vi "3 Optical Motion (Eyes Looking For Geometry).vi"() -> ()   [LabVIEW 2012]
doc: "This example shows how to use the Lucas Kanade Pyramid motion estimation VI to track features in a sequence of images in NI Vision. The VI reads the frames from an AVI file and tracks user specified features in the image from frame to frame."
uses:
  Controls/EyeOptionsCluster.ctl
  <vilib>/userdefined/High Color/IMAQdx.ctl
  <vilib>/vision/Pattern Matching.llb/IMAQ Curve Parameters.ctl
  <vilib>/vision/driver/NI_Vision_Acquisition_Software.lvlib
  <vilib>/vision/NI_Vision_Development_Module.lvlib
panel:
  in  "Eye Options":T1={"Eye Size"=1.0, "Overlay Eyes?"=TRUE, "Eye Tracking?"=TRUE} {"Eye Size" items=["Small"=0.5, "Medium"=1, "Large"=2]}
  in  "Select Points":bool caption="Click on the image and select the points to track. Press the <Ctrl> key while selecting  multiple points. Press the  \"Select Points\" button after  all points have been selected."
  out "Image":T2(plugin-control)
  in  "Stop":bool
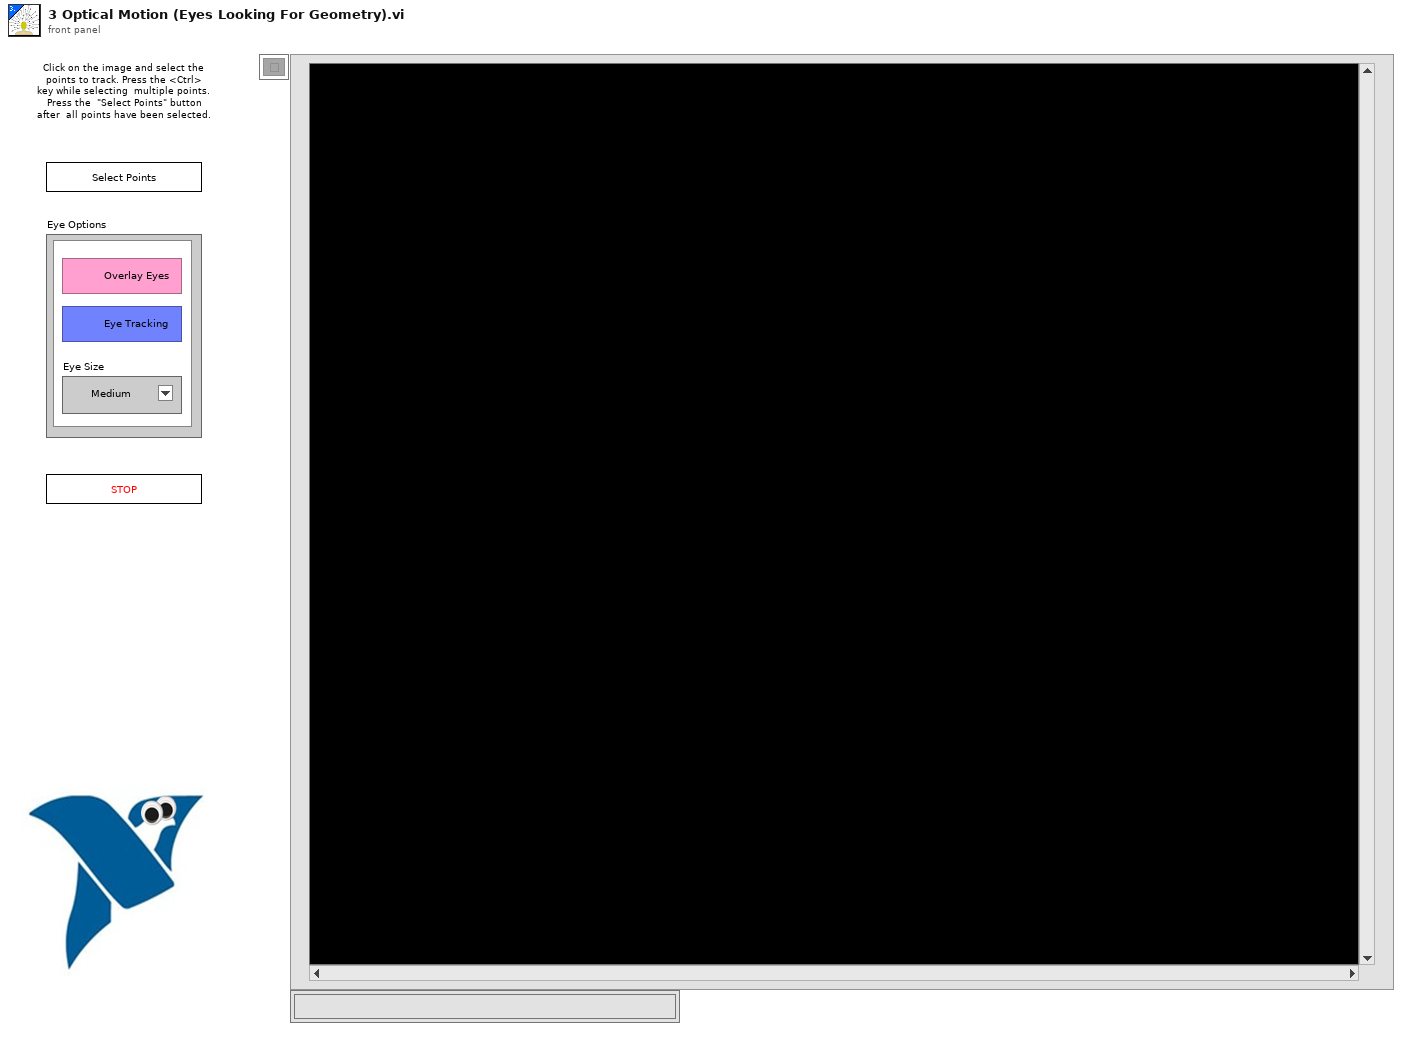
[diagram p1: front panel]
types:
  T1 = typedef "EyeOptionsCluster.ctl" = cluster{"Eye Size":sgl, "Overlay Eyes?":bool, "Eye Tracking?":bool}
  T2 = typedef "IMAQ Image.ctl" = refnum<image>
  T3 = typedef "IMAQ Point" = cluster{"X":sgl, "Y":sgl}
  T4 = typedef "IMAQ Curve Parameters.ctl" = cluster{"Extraction Mode":u32, "Edge Threshold":i32, "Edge Filter Size":u32, "Min Length":i32, "Row Search Step Size":i32, "Col Search Step Size":i32, "Max Endpoint Gap":i32, "Closed":bool, "Subpixel":bool}
  T5 = cluster{"Rotation":bool, "Scale":bool, "Occlusion":bool, "Reserved":bool, "Reserved":bool, "Reserved":bool}
  T6 = typedef "IMAQdx.ctl" = refnum<k21>
  T7 = cluster{"Level":i32, "maxiteration":i32, "windowsize":i32, "threshold":dbl}
  T8 = cluster{"Left":i32, "Top":i32, "Right":i32, "Bottom":i32}
  T9 = typedef "IMAQ GM Match Report.ctl" = cluster{"Position":cluster{"x":sgl, "y":sgl}, "Angle":sgl, "Scale":sgl, "Score":sgl, "Bounding Box":cluster{"x":sgl, "y":sgl}[], "Contrast Reversed":bool, "Occlusion %":sgl, "Template Target Curve Score":sgl, "Target Template Curve Score":sgl, "Correlation Score":sgl}
  T10 = cluster{"Global Rectangle":i32[], "Contours":cluster{"Contour Type":u32, "ROI Type":u32, "Points":i32[]}[]}
  T11 = typedef "ROI Descriptor" = cluster{"Global Rectangle":i32[], "Contours":cluster{"ID":enum32{"External", "Internal"}, "Type":u32, "Coordinates":i32[]}[]}
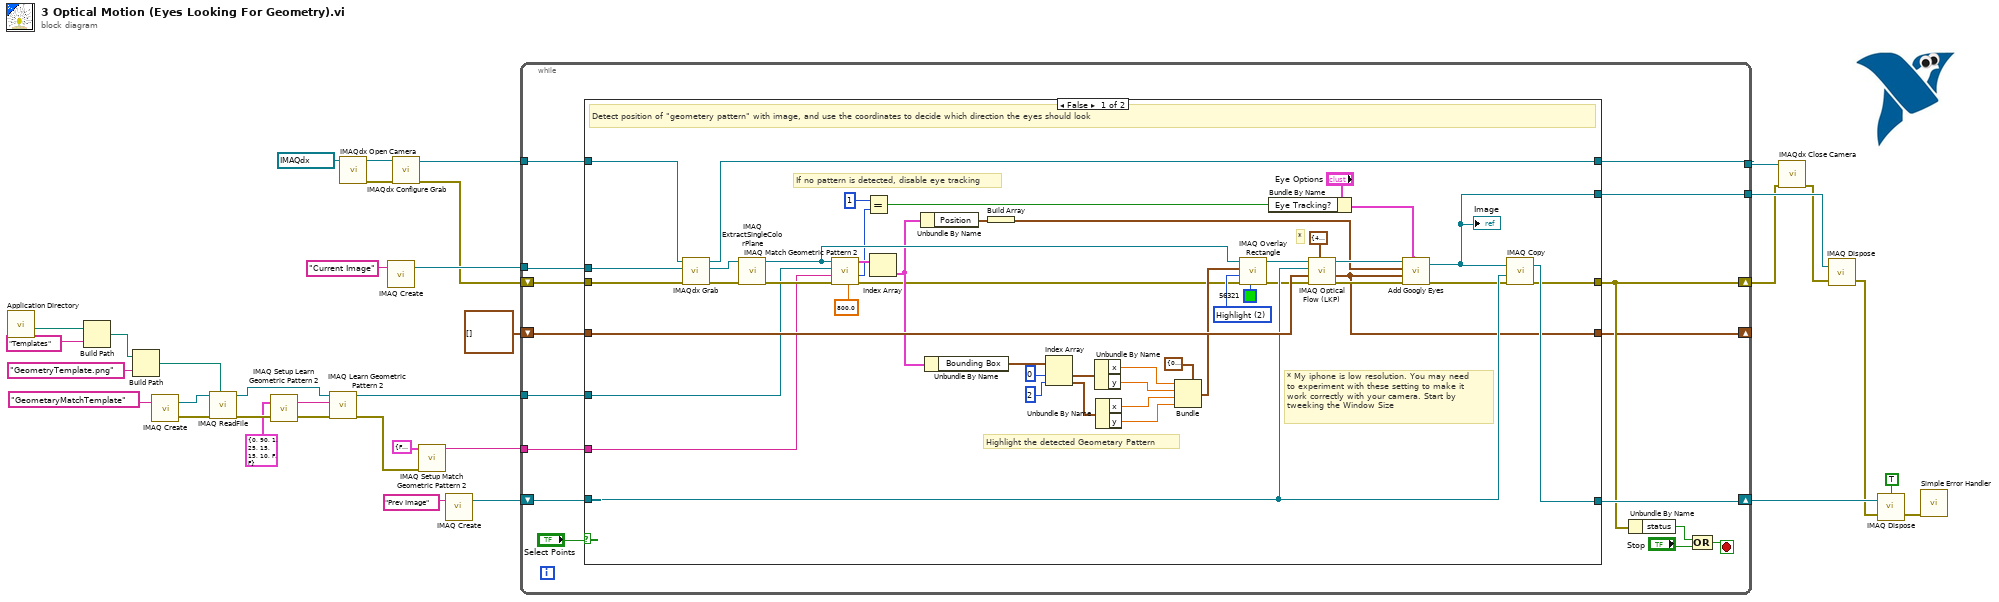
[diagram p0: block diagram]
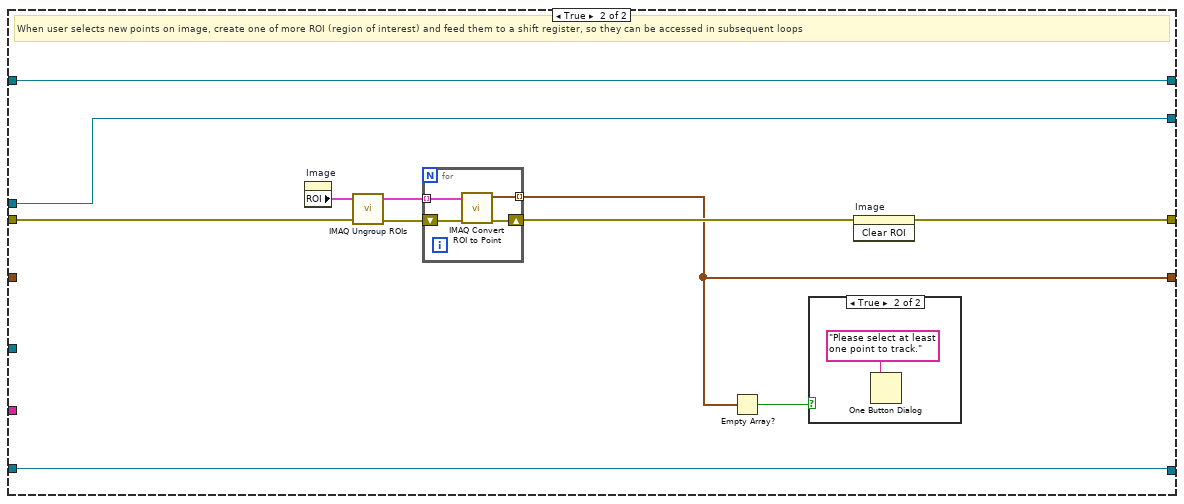
[diagram p2: hidden frame]
diagram:
  n1 = call <vilib>:"Application Directory.vi"() -> ("Application Directory"=w4:path)
  n2 = Build Path(base path=w4, name or relative path="Templates") -> (appended path=w3:path)
  n3 = Build Path(base path=w3, name or relative path="GeometryTemplate.png") -> (appended path=w19:path)
  n4 = call "IMAQ Create"("Image Name"="GeometaryMatchTemplate") -> ("New Image"=w15:T2, "error out"=w17:errorcluster)  [unwired: 4 in]
  n5 = call "IMAQ ReadFile"("File Path"=w19, "error in (no error)"=w17, "Image"=w15) -> ("error out"=w13:errorcluster, "Image Out"=w12:T2)  [unwired: 4 in, 3 out]
  n6 = call "IMAQ Setup Learn Geometric Pattern 2"("error in (no error)"=w13, "Curve Parameters"=T4 {"Extraction Mode"=0, "Edge Threshold"=90, "Edge Filter Size"=1, "Min Length"=25, "Row Search Step Size"=15, "Col Search Step Size"=15, "Max Endpoint Gap"=10, "Closed"=FALSE, "Subpixel"=FALSE}) -> ("error out"=w11:errorcluster, "Learn Geometric Pattern 2 Setup Data"=w9:string)
  n7 = call "IMAQ Learn Geometric Pattern 2"("error in (no error)"=w11, "Learn Geometric Pattern 2 Setup Data"=w9, "Template Image"=w12) -> ("error out"=w7:errorcluster, "Template Image Out"=w10:T2)  [unwired: 7 in]
  n8 = call <vilib>:"IMAQdx Open Camera.vi"("Session In"=T6 "iPhone") -> ("error out"=w27:errorcluster, "Session Out"=w28:T6)  [unwired: 9 in]
  n9 = call "IMAQ Create"("Image Name"="Current Image") -> ("New Image"=w34:T2)  [unwired: 3 in, 2 out]
  n10 = call <vilib>:"IMAQdx Configure Grab.vi"("error in"=w27, "Session In"=w28) -> ("error out"=w21:errorcluster, "Session Out"=w22:T6)  [unwired: 8 in]
  n11 = call "IMAQ Setup Match Geometric Pattern 2"("error in (no error)"=w7, "Match Mode"=T5 {"Rotation"=FALSE, "Scale"=TRUE, "Occlusion"=FALSE, "Reserved"=FALSE, "Reserved"=FALSE, "Reserved"=FALSE}) -> ("Match Geometric Pattern 2 Setup Data"=w8:string)  [unwired: 8 in, 1 out]
  n12 = call "IMAQ Create"("Image Name"="Prev Image") -> ("New Image"=w20:T2)  [unwired: 3 in, 2 out]
  n13 = while {
    tunnel: w34 -> [w41]
    shift-right: [w46] -> w31
    shift-left: w20 -> [w48]
    shift-right: [w43] -> _
    shift-left: T3[] [] ("Feature Points Out") -> [w44]
    shift-right: [w45] -> w26
    shift-left: w21 -> [w51]
    tunnel: [w40] -> w32
    tunnel: w22 -> [w39]
    tunnel: [w38] -> w30
    tunnel: w10 -> [w37]
    tunnel: w8 -> [w36]
    stop <- w49 stop-if-true
    n14 = case shown="False" "Select Points" {
      tunnel: w51 -> [w97 w103]
      tunnel: w41 -> [w96 w102]
      tunnel: w48 -> [w90 w108]
      tunnel: [w95 w108] -> w46
      tunnel: [w94 w99] -> w45
      tunnel: w44 -> [w93 _]
      tunnel: [w84 w101] -> w43
      tunnel: [w83 w102] -> w40
      tunnel: w39 -> [w92 w98]
      tunnel: [w91 w98] -> w38
      tunnel: w37 -> [w80 _]
      tunnel: w36 -> [w79 _]
      frame False {
        w74 = u32 2 items=["Frame", "Fill", "Highlight"] ("Drawing Mode (Frame)")
        # "*"
        # "* My iphone is low resolution. You may need\nto experiment with these setting to make it\nwork correctly with your camera. Start by \ntweeking the Window Size"
        # "Highlight the detected Geometary Pattern"
        # "If no pattern is detected, disable eye tracking"
        # "Detect position of \"geometery pattern\" with image, and use the coordinates to decide which direction the eyes should look"
        n15 = call <vilib>:"IMAQdx Grab.vi"("error in"=w97, "Image In"=w96, "Session In"=w92) -> ("error out"=w87:errorcluster, "Image Out"=w88:T2, "Session Out"=w91:T6)  [unwired: 5 in, 1 out]
        n16 = call "IMAQ ExtractSingleColorPlane"("error in (no error)"=w87, "Image Src"=w88) -> ("error out"=w81:errorcluster, "Image Dst Out"=w73:T2)  [unwired: 8 in]
        n17 = call "IMAQ Match Geometric Pattern 2"("Minimum Match Score"=sgl 800.0, "error in (no error)"=w81, "Match Geometric Pattern 2 Setup Data"=w79, "Template Image"=w80, "Image"=w73) -> ("error out"=w58:errorcluster, "Number of Matches"=w55:i32, "Matches (pixel)"=w77:T9[])  [unwired: 3 in, 1 out]
        n18 = Equal?(x=1, y=w55) -> (x = y?=w53:bool)
        n19 = Index Array(array=w77) -> (element=w64:T9)  [unwired: 1 in]
        n20 = Unbundle By Name(w64) -> ("Position"=w76:cluster{"x":sgl, "y":sgl})
        n21 = Unbundle By Name(w64) -> ("Bounding Box"=w69:cluster{"x":sgl, "y":sgl}[])
        n22 = Build Array(w76) -> (w75:cluster{"x":sgl, "y":sgl}[])
        n23 = Index Array(array=w69, index #1=0 ("index"), index #2=2 ("index")) -> (element #1=w66:cluster{"x":sgl, "y":sgl}, element #2=w65:cluster{"x":sgl, "y":sgl})
        n24 = Unbundle By Name(w66) -> ("x"=w63:sgl, "y"=w62:sgl)
        n25 = Unbundle By Name(w65) -> ("x"=w61:sgl, "y"=w60:sgl)
        n26 = Bundle(cluster=T8 {"Left"=0, "Top"=0, "Right"=0, "Bottom"=0} ("Rectangle"), "Left"=w63, "Top"=w62, "Right"=w61, "Bottom"=w60) -> (w70:T8)
        n27 = call "IMAQ Overlay Rectangle"("Color"=u32 56321, "error in (no error)"=w58, "Drawing Mode (Frame)"=w74, "Rectangle"=w70, "Image"=w73) -> ("error out"=w59:errorcluster, "Image Out"=w72:T2)  [unwired: 5 in]
        n28 = Bundle By Name(cluster="Eye Options", "Eye Tracking?"=w53) -> (w52:T1)
        n29 = call "IMAQ Optical Flow (LKP)"("Options"=T7 {"Level"=4, "maxiteration"=5, "windowsize"=15, "threshold"=0.01} ("Optical Flow Options"), "error in (no error)"=w59, "Feature Points In"=w93, "Previous Frame"=w90, "Current Frame"=w72) -> ("error out"=w86:errorcluster, "Feature Points Out"=w84:cluster{"X":sgl, "Y":sgl}[], "Current Frame Out (dup)"=w82:T2)  [unwired: 1 in, 3 out]
        n30 = call "Add Googly Eyes.vi"("Eye Options"=w52, "error in (no error)"=w86, "Eye Coordinates"=w84, "Feature Coordinates"=w75, "ImageRef In"=w82) -> ("error out"=w89:errorcluster, "ImageRef out"=w83:T2)  [unwired: 5 in]
        "Image" <- w83
        n31 = call "IMAQ Copy"("error in (no error)"=w89, "Image Dst"=w90, "Image Src"=w83) -> ("error out"=w94:errorcluster, "Image Dst Out"=w95:T2)  [unwired: 3 out]
      }
      frame True {
        # "When user selects new points on image, create one of more ROI (region of interest) and feed them to a shift register, so they can be accessed in subsequent loops"
        n32 = property on="Image" class="ImageControl"() -> ("ROI"=w107:T10)  [unwired: 2 in, 2 out]
        n33 = call "IMAQ Ungroup ROIs"("error in (no error)"=w103, "ROI Descriptor"=w107) -> ("error out"=w106:errorcluster, "ROI Descriptors out"=w105:T11[])  [unwired: 2 out]
        n34 = for {
          shift-right: [w110] -> w104
          shift-left: w106 -> [w113]
          tunnel: w105 -> [w112] mode=indexing
          tunnel: [w111] -> w101 mode=indexing
          n35 = call "IMAQ Convert ROI to Point"("error in (no error)"=w113, "ROI Descriptor"=w112) -> ("error out"=w110:errorcluster, "Point"=w111:T3)  [unwired: 7 out]
        }
        n36 = Empty Array?(array=w101) -> (empty?=w100:bool)
        n37 = case shown="True" w100 {
          frame False {
          }
          frame True {
            n38 = One Button Dialog(message="Please select at least one point to track.") -> ()  [unwired: 2 out]
          }
        }
        n39 = invoke on="Image" class="ImageControl" method="Clear ROI"(error in=w104) -> (error out=w99:errorcluster)  [unwired: 2 in, 2 out]
      }
    }
    n40 = Unbundle By Name(w45) -> ("status"=w47:bool)
    n41 = Compound Arithmetic op=OR(w47, "Stop") -> (w49:bool)
  }
  n42 = call <vilib>:"IMAQdx Close Camera.vi"("error in"=w26, "Session In"=w30) -> ("error out"=w25:errorcluster)  [unwired: 9 in]
  n43 = call "IMAQ Dispose"("Image"=w32, "error in (no error)"=w25) -> ("error out"=w24:errorcluster)  [unwired: 1 in, 3 out]
  n44 = call "IMAQ Dispose"("All Images? (No)"=TRUE, "Image"=w31, "error in (no error)"=w24) -> ("error out"=w23:errorcluster)  [unwired: 3 out]
  n45 = call <vilib>:"Simple Error Handler.vi"("error in (no error)"=w23) -> ()  [unwired: 1 in, 8 out]
